vi "Test4.vi"() -> ()   [LabVIEW 2017]
panel:
  out "OutVal":i32
  in  "TrxVal":i32=33
  in  "CSelect":i32=33
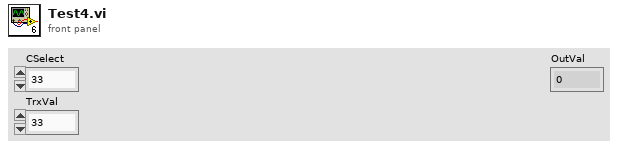
[diagram p1: front panel]
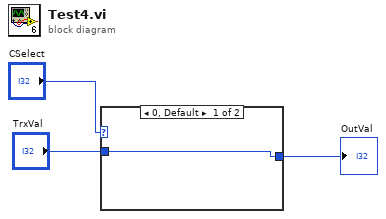
[diagram p0: block diagram]
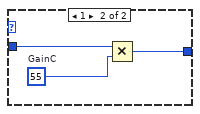
[diagram p2: hidden frame]
diagram:
  n1 = case shown="0, Default" "CSelect" {
    tunnel: "TrxVal" -> [w4 w7]
    tunnel: [w4 w5] -> w1
    frame 0, Default {
    }
    frame 1 {
      w6 = 55  # GainC
      n2 = Multiply(x=w7, y=w6) -> (x*y=w5:i32)
    }
  }
  "OutVal" <- w1
